vi "Wire Release sessions.vi"(0 "Logiv VI Ref":refnum<vi>, 5 "SubVIs Ref":refnum<vi>[](array[refnum]), 11 "error in":errorcluster) -> (15 "error out":errorcluster)   [LabVIEW 2021, in "Migrator.lvlib"]
uses:
  Migrator.lvlib
  Migrator Reusables/Migrator Reusables.lvlib
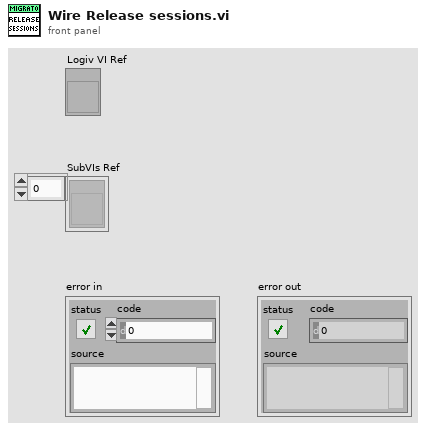
[diagram p1: front panel]
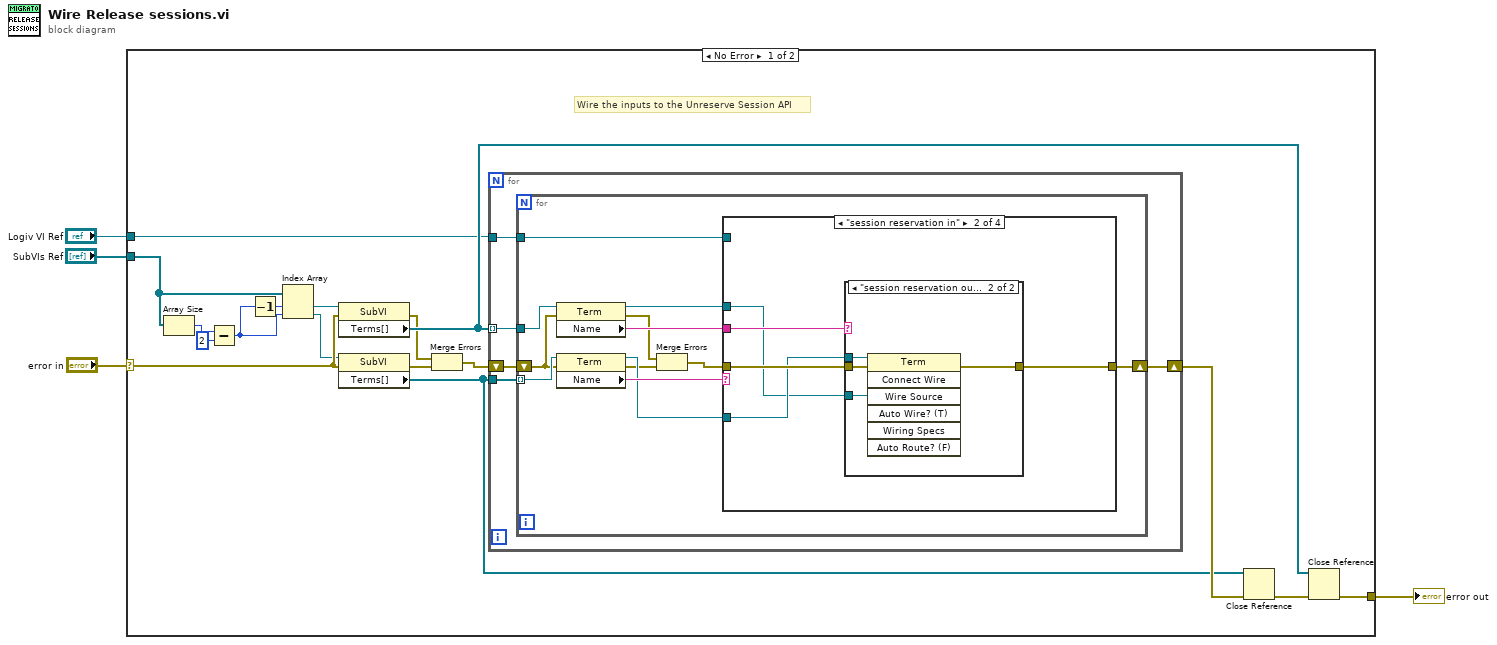
[diagram p0: block diagram]
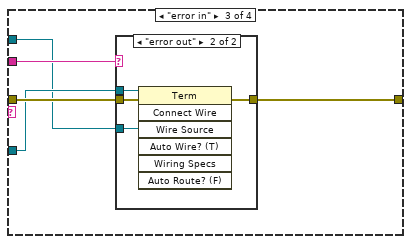
[diagram p4: hidden frame]
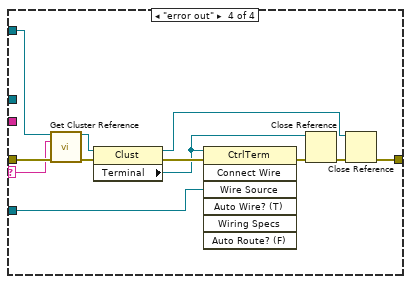
[diagram p6: hidden frame]
diagram:
  n1 = case shown="No Error" "error in" {
    selector: "error in" -> [w21 w72]
    tunnel: [w17 w72] -> w3
    tunnel: "Logiv VI Ref" -> [w12 _]
    tunnel: "SubVIs Ref" -> [w11 _]
    frame No Error {
      # "Wire the inputs to the Unreserve Session API"
      n2 = Array Size(array=w11) -> (size(s)=w8:i32)
      n3 = Subtract(x=w8, y=2) -> (x-y=w6:i32)
      n4 = Decrement(x=w6) -> (x-1=w5:i32)
      n5 = Index Array(array=w11, index #1=w5, index #2=w6) -> (element #1=w14:refnum<vi>, element #2=w13:refnum<vi>)
      n6 = property class="SubVI"(reference=w14, error in=w21) -> (error out=w9:errorcluster, "Terms[]"=w15:refnum<vi>[])  [unwired: 1 out]
      n7 = property class="SubVI"(reference=w13, error in=w21) -> (error out=w20:errorcluster, "Terms[]"=w16:refnum<vi>[])  [unwired: 1 out]
      n8 = Merge Errors(w9, w20) -> (w10:errorcluster)
      n9 = for {
        tunnel: w15 -> [w25] mode=indexing
        tunnel: w16 -> [w26]
        tunnel: w12 -> [w23]
        shift-right: [w22] -> w19
        shift-left: w10 -> [w24]
        n10 = for {
          tunnel: w26 -> [w37] mode=indexing
          tunnel: w25 -> [w38]
          tunnel: w23 -> [w29]
          shift-right: [w30] -> w22
          shift-left: w24 -> [w36]
          n11 = property class="Term"(reference=w38, error in=w36) -> (reference out=w31:refnum<vi>, error out=w27:errorcluster, "Name"=w35:string)
          n12 = property class="Term"(reference=w37, error in=w36) -> (reference out=w33:refnum<vi>, error out=w32:errorcluster, "Name"=w34:string)
          n13 = Merge Errors(w27, w32) -> (w28:errorcluster)
          n14 = case shown="\"session reservation in\"" w34 {
            selector: w34 -> [_ _ _ w69]
            tunnel: w35 -> [_ w44 w54 _]
            tunnel: w33 -> [_ w42 w52 w61]
            tunnel: w28 -> [w39 w43 w53 w70]
            tunnel: [w39 w40 w50 w62] -> w30
            tunnel: w31 -> [_ w41 w51 _]
            tunnel: w29 -> [_ _ _ w71]
            frame Default {
            }
            frame "session reservation in" {
              n15 = case shown="\"session reservation out\"" w44 {
                tunnel: w43 -> [w45 w49]
                tunnel: w42 -> [_ w48]
                tunnel: w41 -> [_ w47]
                tunnel: [w45 w46] -> w40
                frame Default {
                }
                frame "session reservation out" {
                  n16 = invoke class="Term" method="Connect Wire"(reference=w48, error in=w49, "Wire Source"=w47) -> (error out=w46:errorcluster)  [unwired: 4 in, 6 out]
                }
              }
            }
            frame "error in" {
              n17 = case shown="\"error out\"" w54 {
                tunnel: w53 -> [w55 w59]
                tunnel: w52 -> [_ w58]
                tunnel: w51 -> [_ w57]
                tunnel: [w55 w56] -> w50
                frame Default {
                }
                frame "error out" {
                  n18 = invoke class="Term" method="Connect Wire"(reference=w58, error in=w59, "Wire Source"=w57) -> (error out=w56:errorcluster)  [unwired: 4 in, 6 out]
                }
              }
            }
            frame "error out" {
              n19 = call "Get Cluster Reference.vi"("VI in"=w71, "name/order"=w69, "error in (no error)"=w70) -> ("Cluster out"=w65:refnum<vi>, "error out"=w68:errorcluster)  [unwired: 11 in]
              n20 = property class="Clust"(reference=w65, error in=w68) -> (reference out=w60:refnum<vi>, error out=w67:errorcluster, "Terminal"=w66:refnum<vi>)
              n21 = invoke class="CtrlTerm" method="Connect Wire"(reference=w66, error in=w67, "Wire Source"=w61) -> (error out=w64:errorcluster)  [unwired: 4 in, 6 out]
              n22 = Close Reference(reference=w66, error in (no error)=w64) -> (error out=w63:errorcluster)
              n23 = Close Reference(reference=w60, error in (no error)=w63) -> (error out=w62:errorcluster)
            }
          }
        }
      }
      n24 = Close Reference(reference=w16, error in (no error)=w19) -> (error out=w18:errorcluster)
      n25 = Close Reference(reference=w15, error in (no error)=w18) -> (error out=w17:errorcluster)
    }
    frame Error {
    }
  }
  "error out" <- w3
